vi "Parse Sensor Group 1.vi"(11 "stream in":u8[](array[numeric])) -> (1 "Sensor Group 1":T1, 3 "stream out":u8[](array[numeric]))   [LabVIEW 2015]
doc: "Read Sensor Group 1 from a UART data stream."
uses:
  Sensor Group 1.ctl
  Bumps + Wheel Drops.ctl
  Low-Side Driver + Wheel Overcurrent.ctl
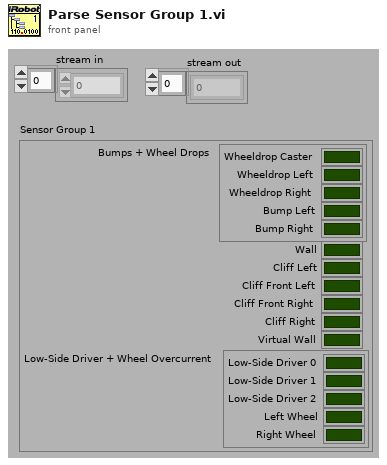
[diagram p1: front panel]
types:
  T1 = typedef "Sensor Group 1.ctl" = cluster{"Bumps + Wheel Drops":T2, "Wall":bool, "Cliff Left":bool, "Cliff Front Left":bool, "Cliff Front Right":bool, "Cliff Right":bool, "Virtual Wall":bool, "Low-Side Driver + Wheel Overcurrent":T3}
  T2 = typedef "Bumps + Wheel Drops.ctl" = cluster{"Wheeldrop Caster":bool, "Wheeldrop Left":bool, "Wheeldrop Right":bool, "Bump Left":bool, "Bump Right":bool}
  T3 = typedef "Low-Side Driver + Wheel Overcurrent.ctl" = cluster{"Low-Side Driver 0":bool, "Low-Side Driver 1":bool, "Low-Side Driver 2":bool, "Left Wheel":bool, "Right Wheel":bool}
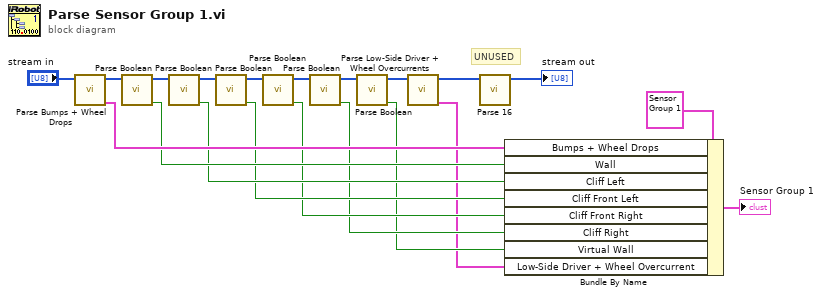
[diagram p0: block diagram]
diagram:
  # "UNUSED"
  n1 = call "Parse Bumps + Wheel Drops.vi"("stream in"="stream in") -> ("Bumps + Wheel Drops"=w10:T2, "stream out"=w19:u8[])  [unwired: 9 out]
  n2 = call "Parse Boolean.vi"("stream in"=w19) -> ("Value"=w9:bool, "stream out"=w18:u8[])  [unwired: 9 out]
  n3 = call "Parse Boolean.vi"("stream in"=w18) -> ("Value"=w8:bool, "stream out"=w17:u8[])  [unwired: 9 out]
  n4 = call "Parse Boolean.vi"("stream in"=w17) -> ("Value"=w7:bool, "stream out"=w16:u8[])  [unwired: 9 out]
  n5 = call "Parse Boolean.vi"("stream in"=w16) -> ("Value"=w6:bool, "stream out"=w15:u8[])  [unwired: 9 out]
  n6 = call "Parse Boolean.vi"("stream in"=w15) -> ("Value"=w5:bool, "stream out"=w14:u8[])  [unwired: 9 out]
  n7 = call "Parse Boolean.vi"("stream in"=w14) -> ("Value"=w4:bool, "stream out"=w13:u8[])  [unwired: 9 out]
  n8 = call "Parse Low-Side Driver + Wheel Overcurrents.vi"("stream in"=w13) -> ("Low-Side Driver + Wheel Overcurrent"=w3:T3, "stream out"=w2:u8[])  [unwired: 9 out]
  n9 = call "Parse 16.vi"("stream in"=w2) -> ("stream out"=→"stream out":u8[])  [unwired: 10 out]
  n10 = Bundle By Name(cluster=T1 {"Bumps + Wheel Drops"={"Wheeldrop Caster"=FALSE, "Wheeldrop Left"=FALSE, "Wheeldrop Right"=FALSE, "Bump Left"=FALSE, "Bump Right"=FALSE}, "Wall"=FALSE, "Cliff Left"=FALSE, "Cliff Front Left"=FALSE, "Cliff Front Right"=FALSE, "Cliff Right"=FALSE, "Virtual Wall"=FALSE, "Low-Side Driver + Wheel Overcurrent"={"Low-Side Driver 0"=FALSE, "Low-Side Driver 1"=FALSE, "Low-Side Driver 2"=FALSE, "Left Wheel"=FALSE, "Right Wheel"=FALSE}} ("Sensor Group 1"), "Bumps + Wheel Drops"=w10, "Wall"=w9, "Cliff Left"=w8, "Cliff Front Left"=w7, "Cliff Front Right"=w6, "Cliff Right"=w5, "Virtual Wall"=w4, "Low-Side Driver + Wheel Overcurrent"=w3) -> (→"Sensor Group 1":T1)
